vi "initialize.vi"(0 "MoAgSy_Visitor_travel":refnum<class "MoAgSy_Visitor_travel.lvclass">, 3 "initializationData":variant, 5 "error in (no error)":errorcluster, 7 "binaryString":string, 8 "I8 Array":i8[](array[numeric]), 9 "prependSize? (T)":bool, 11 "byteOrder (0:big-endian, network order)":T1(ring)) -> (14 "dup MoAgSy_Visitor_travel":refnum<class "MoAgSy_Visitor_travel.lvclass">, 17 "found?":bool, 19 "error out":errorcluster)   [LabVIEW 2009, in "MoAgSy.lvlib" / "MoAgSy_Visitor_travel.lvclass"]
doc: "This is a dynamic dispatch VI to be implemented by child classes to initialize their attributes.\n\n<B>Recommendation:</B> Use Variant for initialization data."
uses:
  MoAgSy_Visitor_travel.lvclass
  MoAgSy_Visitor/MoAgSy_Visitor.lvclass
  MoAgSy_Visitor_travel.lvclass/MoAgSy_Visitor_travel.ctl
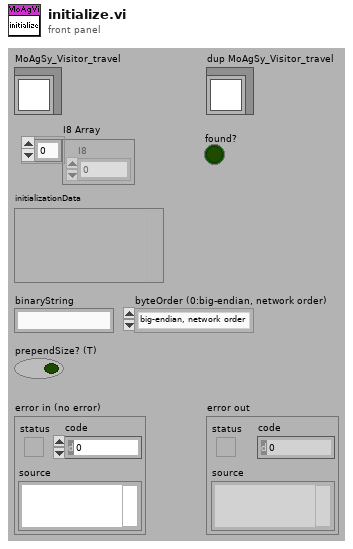
[diagram p1: front panel]
types:
  T1 = enum16{"big-endian, network order", "native, host order", "little-endian"}
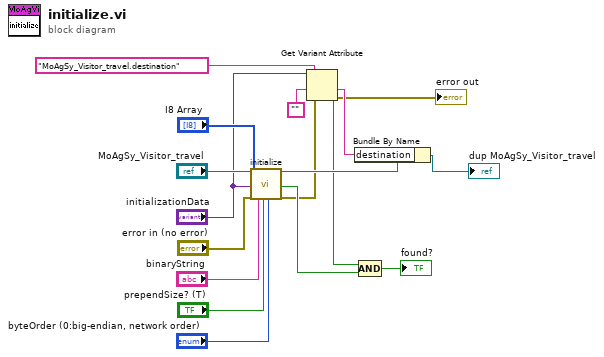
[diagram p0: block diagram]
diagram:
  n1 = call-parent "initialize.vi"("MoAgSy_Visitor"="MoAgSy_Visitor_travel", "initializationData"="initializationData", "error in (no error)"="error in (no error)", "binaryString"="binaryString", "I8 Array"="I8 Array", "prependSize? (T)"="prependSize? (T)", "byteOrder (0:big-endian, network order)"="byteOrder (0:big-endian, network order)") -> ("dup MoAgSy_Visitor"=w11:refnum<class "MoAgSy_Visitor_travel.lvclass">, "found?"=w10:bool, "error out"=w2:errorcluster)  [unwired: 10 out]
  n2 = Get Variant Attribute(Variant="initializationData", name="MoAgSy_Visitor_travel.destination", default value (empty Variant)="", error in=w2) -> (found=w3:bool, value=w5:string, error out=→"error out":errorcluster)  [unwired: 1 out]
  n3 = Bundle By Name(cluster=w11, "destination"=w5) -> (→"dup MoAgSy_Visitor_travel":refnum<class "MoAgSy_Visitor_travel.lvclass">)
  n4 = Compound Arithmetic op=AND(w3, w10) -> (→"found?":bool)
